vi "Test Gantry MPG.vi"() -> ()   [LabVIEW 2011]
uses:
  Gantry Class.lvclass
panel:
  in  "DISABLE":bool
  in  "ENABLE":bool
  in  "Config Folder":path=path "C:/Users/Husker/Desktop/gantry/Config"
  out "error out":errorcluster
  in  "stop":bool
  # "This test is responsible for ensuring the \nfunctionality of the MPG had controller\n***MAKE SURE MOTION COMPOSER IS RUNNING***"
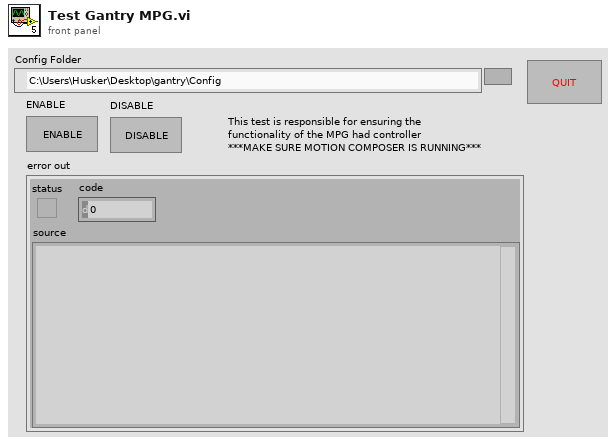
[diagram p1: front panel]
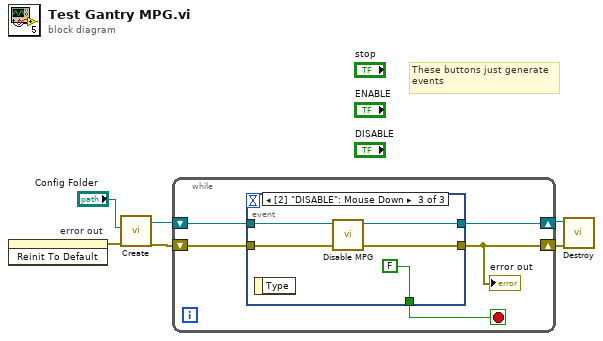
[diagram p0: block diagram]
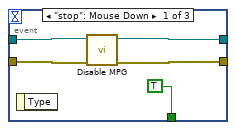
[diagram p2: hidden frame]
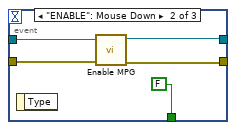
[diagram p3: hidden frame]
diagram:
  # "These buttons just generate\nevents"
  n1 = invoke on="error out" class="Clust (strict)" method="Reinit To Default"() -> (error out=w5:errorcluster)  [unwired: 3 in, 2 out]
  n2 = call "Create.vi"("error in"=w5, "Config Folder"="Config Folder") -> ("error out"=w2:errorcluster, "Gantry out"=w3:refnum<class "Gantry Class.lvclass">)  [unwired: 8 in]
  n3 = while {
    shift-right: [w11] -> w4
    shift-left: w3 -> [w10]
    shift-right: [w7] -> w1
    shift-left: w2 -> [w9]
    stop <- w8 stop-if-true
    n4 = event shown="[2] \"DISABLE\": Mouse Down" {
      selector: _ -> [_ _ _]
      dyn-events: _ -> [_ _ _]
      timeout: _ -> [_ _ _]
      tunnel: w10 -> [w15 w20 w25]
      tunnel: [w16 w18 w24] -> w11
      tunnel: [w13 w17 w22] -> w7
      tunnel: w9 -> [w14 w19 w23]
      tunnel: [TRUE FALSE FALSE] -> w8
      event "stop": Mouse Down {
        n5 = event-data() -> ()  [unwired: 1 in, 1 out]
        n6 = call-dynamic "Disable MPG.vi"("error in (no error)"=w14, "Gantry Class in"=w15) -> ("error out"=w13:errorcluster, "Gantry Class out"=w16:refnum<class "Gantry Class.lvclass">)  [unwired: 8 in]
      }
      event "ENABLE": Mouse Down {
        n7 = event-data() -> ()  [unwired: 1 in, 1 out]
        n8 = call-dynamic "Enable MPG.vi"("error in (no error)"=w19, "Gantry Class in"=w20) -> ("error out"=w17:errorcluster, "Gantry Class out"=w18:refnum<class "Gantry Class.lvclass">)  [unwired: 8 in]
      }
      event "DISABLE": Mouse Down {
        n9 = event-data() -> ()  [unwired: 1 in, 1 out]
        n10 = call-dynamic "Disable MPG.vi"("error in (no error)"=w23, "Gantry Class in"=w25) -> ("error out"=w22:errorcluster, "Gantry Class out"=w24:refnum<class "Gantry Class.lvclass">)  [unwired: 8 in]
      }
    }
    "error out" <- w7
  }
  n11 = call "Destroy.vi"("error in"=w1, "Gantry Class in"=w4) -> ()  [unwired: 9 in, 1 out]
